vi "CLD3 FGV Timer no pause solution.vi"(8 "Fehler (Eingang, kein Fehler)":errorcluster, 10 "Warten":dbl, 11 "Timer-Task":T1) -> (0 "Fehler (Ausgang)":errorcluster, 2 "Verstrichene Zeit?":bool, 3 "Verstrichene Zeit":dbl)   [LabVIEW 2014]
doc: "CLD-Zusatzaufgabe 3\n\nEinfache Messung der verstrichenen Zeit. Ermittelt die Zeitdifferenz in Sekunden mit Hilfe eines Zeitstempelvergleichs."
uses:
  CLD3 Timer Mode.ctl
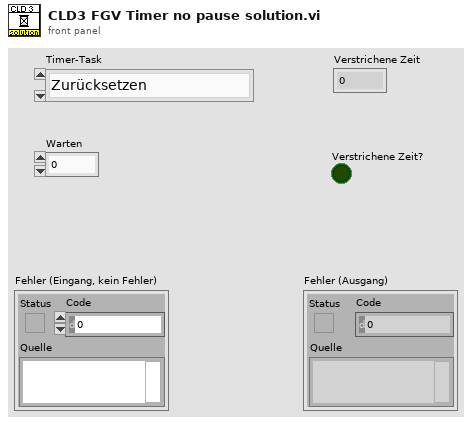
[diagram p1: front panel]
types:
  T1 = typedef "CLD3 Timer Mode.ctl" = enum16{"Zurücksetzen", "Verstrichen"}
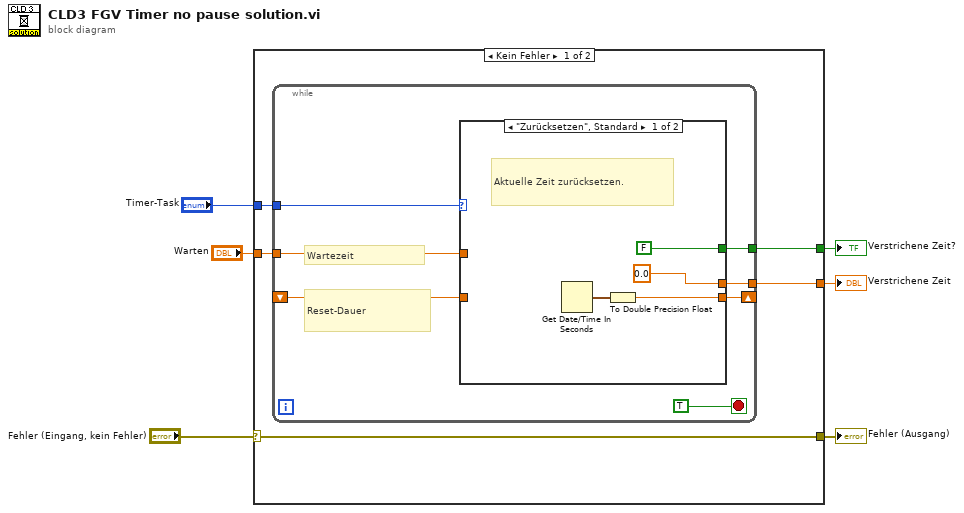
[diagram p0: block diagram]
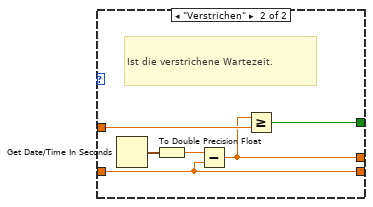
[diagram p2: hidden frame]
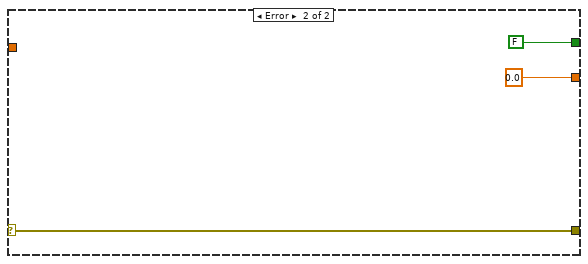
[diagram p3: hidden frame]
diagram:
  n1 = case shown="Kein Fehler" "Fehler (Eingang, kein Fehler)" {
    selector: "Fehler (Eingang, kein Fehler)" -> [w8 w31]
    tunnel: "Timer-Task" -> [w11 _]
    tunnel: "Warten" -> [w10 _]
    tunnel: [w9 FALSE] -> w5
    tunnel: [w8 w31] -> w3
    tunnel: [w7 0.0] -> w2
    frame No Error {
      n2 = while {
        tunnel: w11 -> [w17]
        shift-right: [w16] -> _
        shift-left: _ -> [w15]
        tunnel: w10 -> [w14]
        tunnel: [w13] -> w9
        tunnel: [w12] -> w7
        stop <- TRUE stop-if-true
        # "Reset-Dauer"
        # "Wartezeit"
        n3 = case shown="\"Zurücksetzen\", Standard" w17 {
          tunnel: [w21 w23] -> w16
          tunnel: w15 -> [_ w23]
          tunnel: w14 -> [_ w27]
          tunnel: [FALSE w26] -> w13
          tunnel: [0.0 w25] -> w12
          frame "Zurücksetzen", Default {
            # "Aktuelle Zeit zurücksetzen."
            n4 = Get Date/Time In Seconds() -> (seconds since 1Jan1904=w22:timestamp)
            n5 = To Double Precision Float(number=w22) -> (double precision float=w21:dbl)
          }
          frame "Verstrichen" {
            # "Ist die verstrichene Wartezeit."
            n6 = Get Date/Time In Seconds() -> (seconds since 1Jan1904=w28:timestamp)
            n7 = To Double Precision Float(number=w28) -> (double precision float=w24:dbl)
            n8 = Subtract(x=w24, y=w23) -> (x-y=w25:dbl)
            n9 = Greater Or Equal?(x=w25, y=w27) -> (x >= y?=w26:bool)
          }
        }
      }
    }
    frame Error {
    }
  }
  "Verstrichene Zeit?" <- w5
  "Fehler (Ausgang)" <- w3
  "Verstrichene Zeit" <- w2
